vi "Set Magnet Field.vi"(4 "Axis":T1, 6 "Mode":T2, 8 "error in (no error)":errorcluster, 9 "Target Rate (T/min)":dbl, 10 "Target Field (T)":dbl, 11 "Instrument.Oxford1820 in":refnum<class "Instrument.Oxford1820.lvclass">) -> (0 "error out":errorcluster, 3 "Instrument.Oxford1820 out":refnum<class "Instrument.Oxford1820.lvclass">)   [LabVIEW 2016, in "Instrument.Oxford1820.lvclass"]
uses:
  Instrument.Oxford1820.lvclass
  <userlib>/LevyLab/Levylab Instruments/Instrument Types/Cryostat/Typedefs/Magnet Mode--Enum.ctl
  <userlib>/LevyLab/Levylab Instruments/Instrument Types/Cryostat/Typedefs/Magnet Axis--Enum.ctl
  Typedefs/Targets.ctl
  <userlib>/LevyLab/Levylab Instruments/Instrument Types/Cryostat/Instrument.Cryostat.lvclass
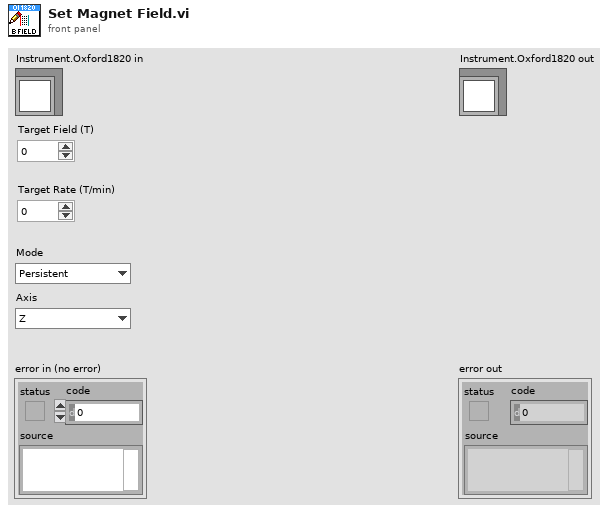
[diagram p1: front panel]
types:
  T1 = typedef "Instrument.Cryostat.lvclass/Magnet Axis--Enum.ctl" = enum16{"Z", "X", "Y"}
  T2 = typedef "Instrument.Cryostat.lvclass/Magnet Mode--Enum.ctl" = enum16{"Persistent", "Driven"}
  T3 = typedef "Targets.ctl" = cluster{"Target Field (T)":dbl, "Target Field Rate (T/min)":dbl}
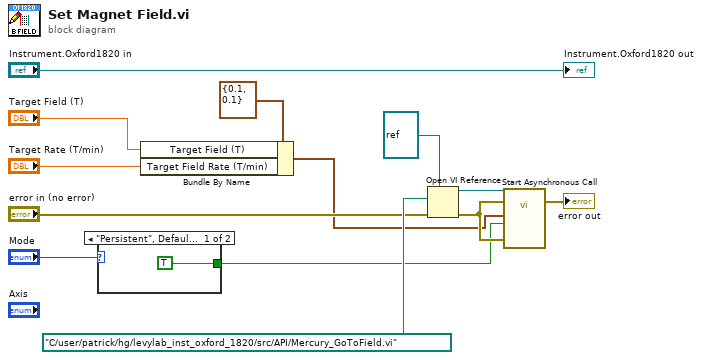
[diagram p0: block diagram]
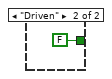
[diagram p2: hidden frame]
diagram:
  n1 = case shown="\"Persistent\", Default" "Mode" {
    tunnel: [TRUE ("persistent mode") FALSE ("persistent mode")] -> w2
    frame "Persistent", Default {
    }
    frame "Driven" {
    }
  }
  n2 = Bundle By Name(cluster=T3 {"Target Field (T)"=0.1, "Target Field Rate (T/min)"=0.1} ("Mercury Targets"), "Target Field (T)"="Target Field (T)", "Target Field Rate (T/min)"="Target Rate (T/min)") -> (w1:T3)
  n3 = Open VI Reference(type specifier VI Refnum (for type only)=refnum<vi> refnum, vi path=path "C:/user/patrick/hg/levylab_inst_oxford_1820/src/API/Mercury_GoToField.vi", error in (no error)="error in (no error)") -> (vi reference=w7:refnum<vi>, error out=w3:errorcluster)  [unwired: 3 in]
  n4 = call-by-ref "Start Asynchronous Call"(reference=w7, error in=w3, "error in"=w3, "persistent mode"=w2, "Mercury Targets"=w1) -> (error out=→"error out":errorcluster)  [unwired: 8 in, 2 out]
  "Instrument.Oxford1820 out" <- "Instrument.Oxford1820 in"
